vi "Execution Start.vi"(7 "Execution Data":variant, 8 "error in (no error)":errorcluster, 11 "Execution in":refnum<data-value>) -> (0 "error out":errorcluster, 3 "Execution out":refnum<data-value>)   [LabVIEW 2015, in "Execution.lvclass"]
uses:
  Execution.lvclass
  EXECUTION_STATUS.ctl
  EXECUTION_CTRL_MSG.ctl
  STEP_CONTEXT.ctl
  Step.lvclass
  Step/STEP_STATUS.ctl
  EXECUTION_UI_MSG.ctl
  EXECUTION_RESULT_TYPEDEF.ctl
  STEP_RESULT.ctl
  STEP_MEASURE_RESULT.ctl
  Step/OUTPUT_DATA_TYPE.ctl
  OutputUI/OUTPUT_CHECK_TYPE.ctl
  Send UI Message.vi
  Send Control Message.vi
  Project.lvclass
  Plugin.lvclass
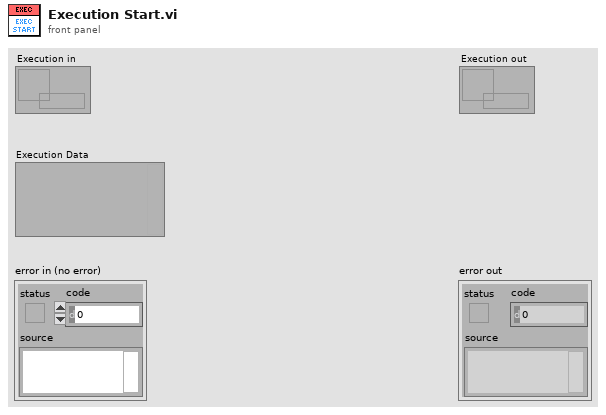
[diagram p1: front panel]
types:
  T1 = typedef "Execution.lvclass/STEP_RESULT.ctl" = cluster{"StepIndex":u32, "Step":refnum<class "Step.lvclass">, "StartTime":timestamp, "EndTime":timestamp, "Result":T2, "Error Info":string, "Measure Results":T3[]}
  T2 = typedef "Step.lvclass/STEP_STATUS.ctl" = enum16{"Skipped", "Done", "Passed", "Failed", "Error"}
  T3 = typedef "Execution.lvclass/STEP_MEASURE_RESULT.ctl" = cluster{"Name":string, "Data Type":T4, "Check Type":T5, "String Limit":string, "Lower Limit":dbl, "Upper Limit":dbl, "Boolean Limit":bool, "Ignore Case":bool, "Measure Data":variant, "Result":T2, "Error Info":string}
  T4 = typedef "Step.lvclass/OUTPUT_DATA_TYPE.ctl" = enum16{"Boolean", "String", "Numeric", "Other"}
  T5 = typedef "Step.lvclass/OUTPUT_CHECK_TYPE.ctl" = enum16{"INVALID", "DO_NOT_CHECK", "RECORD", "VARIABLE", "EQUAL", "NOT_EQUAL", "STR_CONTAINS", "STR_START_WITH", "STR_END_WITH", "STR_REGEX_MATCH", "NUM_GT", "NUM_LT", "NUM_GE", "NUM_LE", "NUM_RANGE", "NUM_RANGE_BDY"}
  T6 = typedef "Execution.lvclass/EXECUTION_RESULT_TYPEDEF.ctl" = enum16{"Unknow", "Terminated", "Passed", "Failed", "Error"}
  T7 = typedef "Execution.lvclass/EXECUTION_UI_MSG.ctl" = enum16{"EXECUTION_STATUS", "INIT_UI", "DUT_UPDATE", "BOTTOM_PANEL_UPDATE", "TOP_PANEL_UPDATE", "STEP_START", "STEP_END", "DISPLAY_RESULT", "APPLICATION_END"}
  T8 = typedef "Execution.lvclass/STEP_CONTEXT.ctl" = cluster{"StepIndex":u32, "Step":refnum<class "Step.lvclass">, "StartTime":timestamp, "EndTime":timestamp, "Result":T2, "Error Info":string, "Output Values":cluster{"Name":string, "Variant Data":variant}[]}
  T9 = typedef "Execution.lvclass/EXECUTION_CTRL_MSG.ctl" = enum16{"EXECUTION_START", "EXECUTION_END", "EXECUTION_LOOP", "APPLICATION_STOP"}
  T10 = typedef "Execution.lvclass/EXECUTION_STATUS.ctl" = enum16{"Initializing ", "Disable", "Ready", "Running", "Finished"}
  T11 = typedef "DUT_INFO_TYPEDEF.ctl" = cluster{"SN":string, "Model":string, "PartNumber":string, "Revision":string, "Software":string, "Hardware":string}
  T12 = typedef "Execution.lvclass/EXECUTION_CONTEXT.ctl" = cluster{"Continue Test":bool, "DUT Info":T13, "StartTime":timestamp, "EndTime":timestamp, "Result":T6, "Info Text":string, "ResultList":T1[]}
  T13 = typedef "Execution.lvclass/DUT_INFO_TYPEDEF.ctl" = cluster{"SN":string, "Model":string, "PartNumber":string, "Revision":string, "Software":string, "Hardware":string}
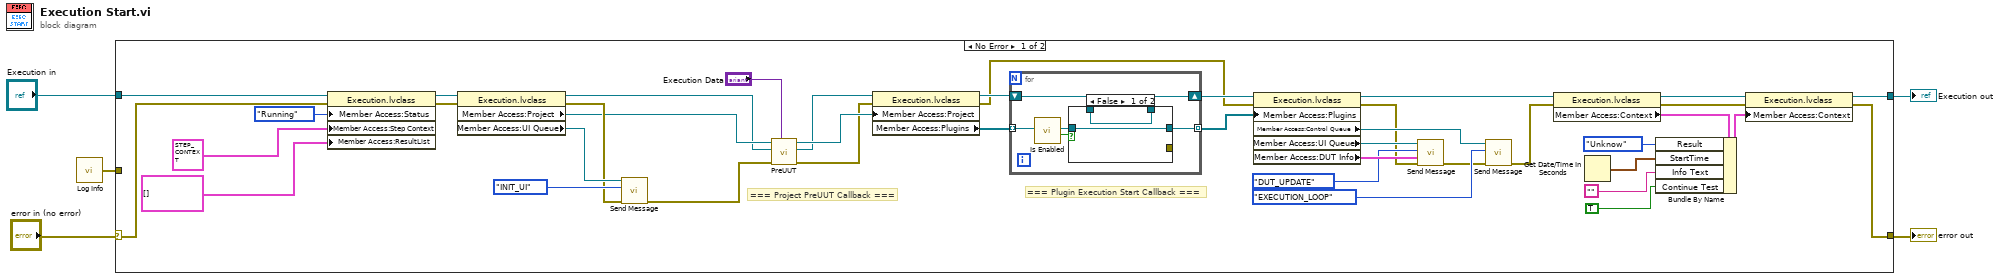
[diagram p0: block diagram]
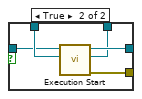
[diagram p2: hidden frame]
diagram:
  n1 = call "Log Info.vi"() -> ("error out"=w1:errorcluster)  [unwired: 5 in]
  n2 = case shown="No Error" "error in (no error)" {
    selector: "error in (no error)" -> [w42 w61]
    tunnel: [w13 w61] -> w4
    tunnel: [w15 w60] -> w2
    tunnel: "Execution in" -> [w41 w60]
    tunnel: w1 -> [_ _]
    frame No Error {
      # "=== Project PreUUT Callback ==="
      # "=== Plugin Execution Start Callback ==="
      n3 = property class="Execution.lvclass"(reference=w41, error in=w42, "Member Access:Status"=EXECUTION_STATUS."Running" ("Status"), "Member Access:Step Context"=T8 {"StepIndex"=0, "Step"=refnum, "StartTime"=timestamp(0 s since 1904-01-01), "EndTime"=timestamp(0 s since 1904-01-01), "Result"=enum."Skipped", "Error Info"="", "Output Values"=[]} ("Context"), "Member Access:ResultList"=T1[] [] ("ResultList")) -> (reference out=w39:refnum<data-value>, error out=w40:errorcluster)
      n4 = property class="Execution.lvclass"(reference=w39, error in=w40) -> (reference out=w27:refnum<data-value>, error out=w37:errorcluster, "Member Access:Project"=w36:refnum<class "Project.lvclass">, "Member Access:UI Queue"=w38:refnum<queue>)
      n5 = call-poly "Send Message.vi"("error in (no error)"=w37, "Msg"=EXECUTION_UI_MSG."INIT_UI", "UI Queue"=w38) -> ("error out"=w24:errorcluster)  [unwired: 8 in]
      n6 = call-dynamic "PreUUT.vi"("Execution Data"="Execution Data", "error in (no error)"=w24, "Execution in"=w27, "TestProjectBase in"=w36) -> ("error out"=w34:errorcluster, "Execution out"=w26:refnum<data-value>, "TestProjectBase out"=w35:refnum<class "Project.lvclass">)  [unwired: 5 in]
      n7 = property class="Execution.lvclass"(reference=w26, error in=w34, "Member Access:Project"=w35) -> (reference out=w32:refnum<data-value>, error out=w29:errorcluster, "Member Access:Plugins"=w33:refnum<class "Plugin.lvclass">[])
      n8 = for {
        tunnel: w33 -> [w49] mode=indexing
        shift-right: [w50] -> w31
        shift-left: w32 -> [w51]
        tunnel: [w52] -> w30 mode=indexing
        n9 = call "Is Enabled.vi"("Plugin in"=w49) -> ("Enabled"=w47:bool, "Plugin out"=w48:refnum<class "Plugin.lvclass">)  [unwired: 9 in]
        n10 = case shown="False" w47 {
          tunnel: [w53 w59] -> w52
          tunnel: [_ w58] -> _
          tunnel: w51 -> [w54 w57]
          tunnel: [w54 w56] -> w50
          tunnel: w48 -> [w53 w55]
          frame False {
          }
          frame True {
            n11 = call-dynamic "Execution Start.vi"("Execution in"=w57, "Plugin in"=w55) -> ("error out"=w58:errorcluster, "Execution out"=w56:refnum<data-value>, "Plugin out"=w59:refnum<class "Plugin.lvclass">)  [unwired: 7 in]
          }
        }
      }
      n12 = property class="Execution.lvclass"(reference=w31, error in=w29, "Member Access:Plugins"=w30) -> (reference out=w17:refnum<data-value>, error out=w20:errorcluster, "Member Access:Control Queue"=w28:refnum<queue>, "Member Access:UI Queue"=w23:refnum<queue>, "Member Access:DUT Info"=w22:T11)
      n13 = call-poly "Send Message.vi"("error in (no error)"=w20, "Data"=w22, "Msg"=EXECUTION_UI_MSG."DUT_UPDATE", "UI Queue"=w23) -> ("error out"=w19:errorcluster)  [unwired: 7 in]
      n14 = call-poly "Send Message.vi"("error in (no error)"=w19, "Msg"=EXECUTION_CTRL_MSG."EXECUTION_LOOP", "Control Queue"=w28) -> ("error out"=w18:errorcluster)  [unwired: 8 in]
      n15 = property class="Execution.lvclass"(reference=w17, error in=w18) -> (reference out=w16:refnum<data-value>, error out=w14:errorcluster, "Member Access:Context"=w9:T12)
      n16 = Get Date/Time In Seconds() -> (seconds since 1Jan1904=w11:timestamp)
      n17 = Bundle By Name(cluster=w9, "Result"=EXECUTION_RESULT_TYPEDEF."Unknow", "StartTime"=w11, "Info Text"="", "Continue Test"=TRUE) -> (w8:T12)
      n18 = property class="Execution.lvclass"(reference=w16, error in=w14, "Member Access:Context"=w8) -> (reference out=w15:refnum<data-value>, error out=w13:errorcluster)
    }
    frame Error {
    }
  }
  "error out" <- w4
  "Execution out" <- w2
